vi "uObserver_Set_DoesOwnBroker.vi"(8 "error in (no error)":errorcluster, 10 "DoesOwnBroker?":bool=TRUE, 11 "uObserver in":refnum<class "uObserver.lvclass">) -> (0 "error out":errorcluster, 3 "uObserver out":refnum<class "uObserver.lvclass">)   [LabVIEW 2023, in "uLib.lvlib" / "uObserver.lvclass"]
doc: "In general, when a non-observer actor attempts to launch an observer actor, an error will occur at the caller. The reason is that the caller will fail to process the request from the callee to provide the transport of the common observed broker.\n\nUse this accessor method when a non-observer actor attempts to launch an observer actor. The callee here is instructed to launch its own broker and cascade it down to its own callees throughout that hierarchy which is managed by the observer. So the callee does own its own broker.\n\nDo NOT use this method in conjunction with the Set_Broker accessor method."
uses:
  uObserver.lvclass
  uObserver.lvclass/uObserver.ctl
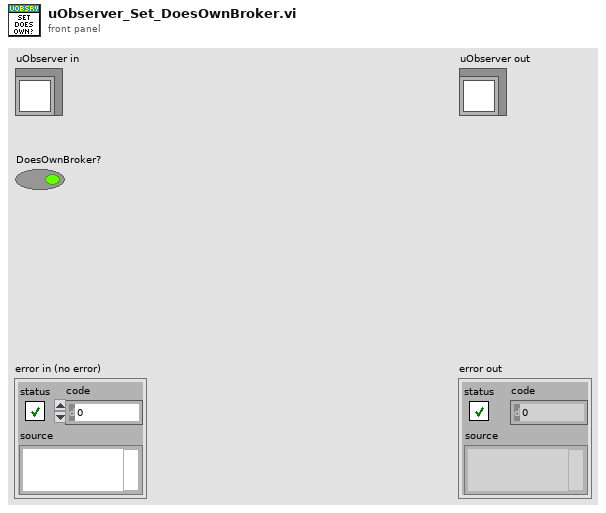
[diagram p1: front panel]
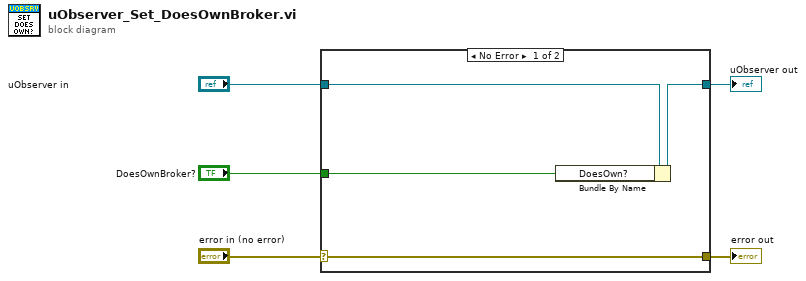
[diagram p0: block diagram]
diagram:
  n1 = case shown="No Error" "error in (no error)" {
    selector: "error in (no error)" -> [w9 w10]
    tunnel: [w9 w10] -> w4
    tunnel: [w7 w11] -> w2
    tunnel: "uObserver in" -> [w8 w11]
    tunnel: "DoesOwnBroker?" -> [w6 _]
    frame No Error {
      n2 = Bundle By Name(cluster=w8, "DoesOwn?"=w6) -> (w7:refnum<class "uObserver.lvclass">)
    }
    frame Error {
    }
  }
  "error out" <- w4
  "uObserver out" <- w2
